vi "VG-format_for_smith.vi"() -> ()   [LabVIEW 2020, in "VG-VNA_GUI.lvlib" / "VG-VNA_GUI.lvclass"]
uses:
  VG-VNA_GUI.lvclass
  VG-graph_data.ctl
  <vilib>/picture/smith.llb/Smith Plot Style.ctl
panel:
  out "Array":cluster{dbl, dbl}[](array[cluster])
  out "XY Graph 3":cluster{u64[], dbl[]}[](graph)
  in  "smith grid cosmetics":T1={"R color"=8355711, "R grids"=TRUE, "X color"=5000268, "X grids"=TRUE, "Labels"=TRUE}
  in  "smith plot cosmetics":T3={"Plot Style"=2, "Line Color"=39423, "Point Color"=39423} {"Plot Style" items=["Points", "Lines", "Lines & Points"]}
  in  "smith plot section":T4={"x minimum"=-1.0, "x maximum"=1.0, "y minimum"=-1.0, "y maximum"=1.0} {"x minimum" format="%0.2f"; "x maximum" format="%0.2f"; "y minimum" format="%0.2f"; "y maximum" format="%0.2f"}
  in  "top left point(0, 0)":cluster{"x":i16, "y":i16}
  in  "dimensions incl scales? (T)":bool=TRUE
  in  "[user-specified font]":T5
  in  "desired font(Application)":T6(ring)=enum."Application Font"
  out "Smith Plot":picture
  in  "Graph Data":T7
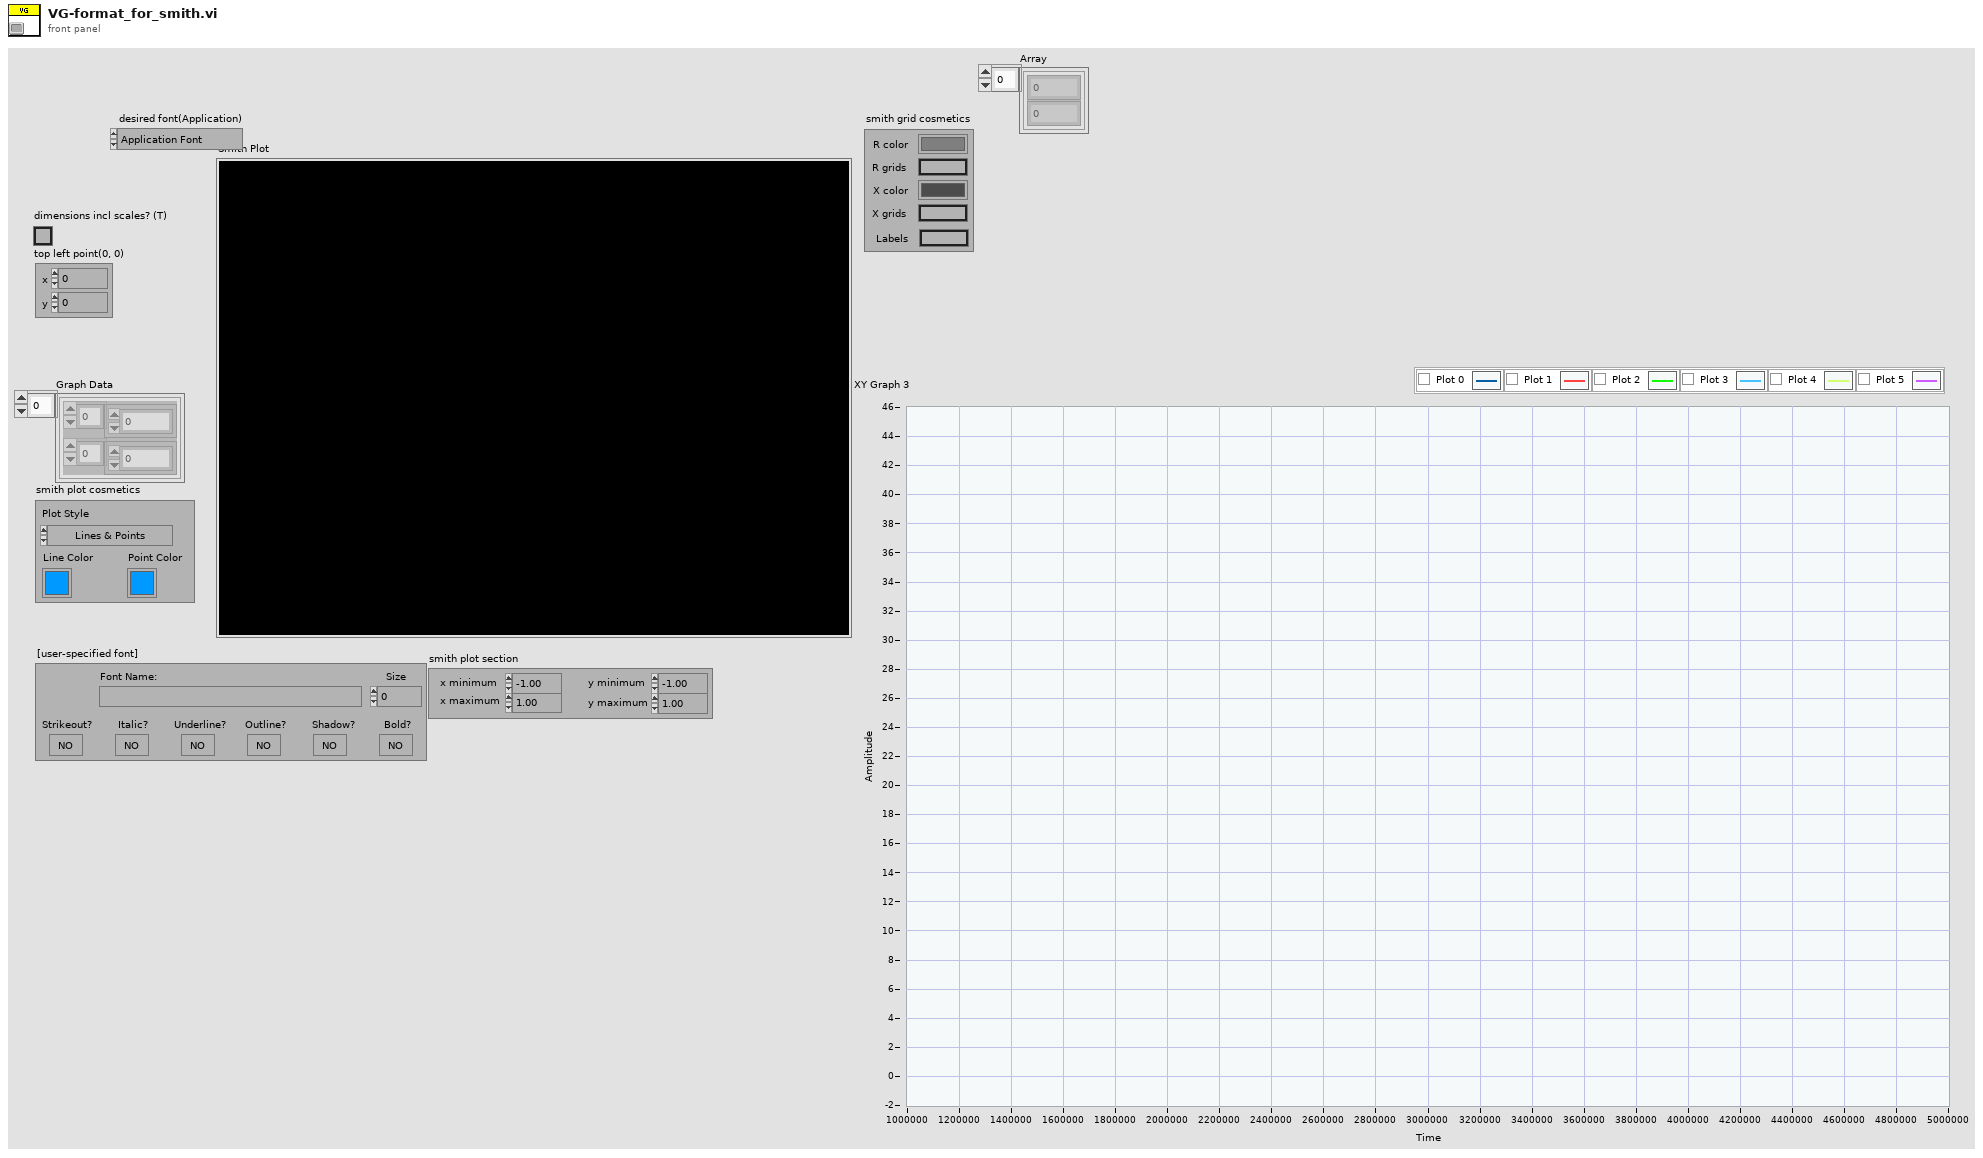
[diagram p1: front panel]
types:
  T1 = cluster{"R color":u32, "R grids":bool, "X color":u32, "X grids":bool, "Labels":bool}
  T2 = typedef "Smith Plot Style.ctl" = u16
  T3 = cluster{"Plot Style":T2, "Line Color":u32, "Point Color":u32}
  T4 = cluster{"x minimum":dbl, "x maximum":dbl, "y minimum":dbl, "y maximum":dbl}
  T5 = cluster{"Font Name:":string, "Size":i16, "Strikeout?":bool, "Italic?":bool, "Underline?":bool, "Outline?":bool, "Shadow?":bool, "Bold?":bool}
  T6 = enum16{"User-specified Font", "Application Font", "System Font", "Dialog Font"}
  T7 = typedef "VG-VNA_GUI.lvlib/VG-VNA_GUI.lvclass/VG-graph_data.ctl" = cluster{u64[], dbl[]}[]
  T8 = typedef "LVBoundsTypeDef.ctl" = cluster{"Width":u32, "Height":u32}
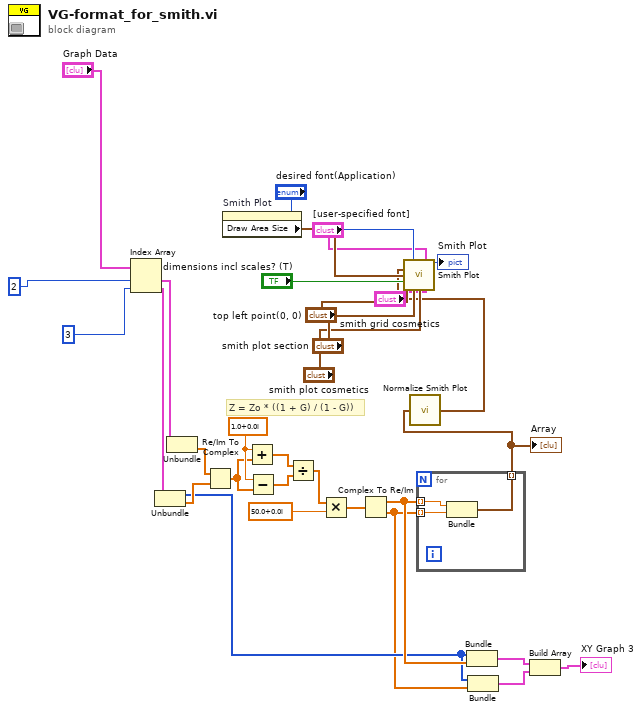
[diagram p0: block diagram]
diagram:
  w24 = cdb 1.0+0.0i ("x")
  # "Z = Zo * ((1 + G) / (1 - G))"
  n1 = Index Array(array="Graph Data", index #1=2 ("index"), index #2=3 ("index")) -> (element #1=w27:cluster{u64[], dbl[]}, element #2=w26:cluster{u64[], dbl[]})
  n2 = Unbundle(w26) -> (w7:u64[], w17:dbl[])
  n3 = Unbundle(w27) -> (w16:dbl[])  [unwired: 1 out]
  n4 = Re/Im To Complex(1:w17, 2:w16) -> (0:w18:cdb[])
  n5 = property on="Smith Plot" class="Pict"() -> ("Draw Area Size"=w30:T8)  [unwired: 2 in, 2 out]
  n6 = Add(x=w24, y=w18) -> (x+y=w23:cdb[])
  n7 = Subtract(x=w24, y=w18) -> (x-y=w22:cdb[])
  n8 = Divide(x=w23, y=w22) -> (x/y=w21:cdb[])
  n9 = Multiply(x=w21, y=cdb 50.0+0.0i) -> (x*y=w19:cdb[])
  n10 = Complex To Re/Im(x + iy=w19) -> (x=w8:dbl[], y=w6:dbl[])
  n11 = for {
    tunnel: w8 -> [w34] mode=indexing
    tunnel: w6 -> [w33] mode=indexing
    tunnel: [w32] -> w2 mode=indexing
    n12 = Bundle(w34, w33) -> (w32:cluster{dbl, dbl})  [unwired: 1 in]
  }
  "Array" <- w2
  n13 = call <vilib>:"Normalize Smith Plot.vi"("points {r,x}"=w2) -> ("normalized smith points {r,x}"=w1:cluster{"r":dbl, "x":dbl}[])  [unwired: 2 in]
  n14 = call <vilib>:"Smith Plot.vi"("desired font(Application)"="desired font(Application)", "[user-specified font]"="[user-specified font]", "smith plot"=w1, "dimensions (w,h)"=w30, "dimensions incl scales? (T)"="dimensions incl scales? (T)", "top left point(0, 0)"="top left point(0, 0)", "smith plot section"="smith plot section", "smith plot cosmetics"="smith plot cosmetics", "smith grid cosmetics"="smith grid cosmetics") -> ("new picture"=→"Smith Plot":picture)  [unwired: 6 in]
  n15 = Bundle(w7, w8) -> (w5:cluster{u64[], dbl[]})  [unwired: 1 in]
  n16 = Bundle(w7, w6) -> (w4:cluster{u64[], dbl[]})  [unwired: 1 in]
  n17 = Build Array(w5, w4) -> (→"XY Graph 3":cluster{u64[], dbl[]}[])
